vi "Event Handler.vi"(8 "error in (no error)":errorcluster, 10 "Stop Event Handler":refnum<user-event>, 11 "BreadcrumbNavigation in":refnum<class "BreadcrumbNavigator.lvclass">) -> (0 "error out":errorcluster)   [LabVIEW 2015, in "BreadcrumbNavigator.lvclass"]
doc: "The <b>Event Handler VI</b> is a dynamic dispatch VI that should be overwritten if events are needed to create the enhanced QControl. \n\nBy inheriting from the main Control.lvclass the overwritten <b>Event Handler VI</b> will be launched asynchronously in the initialization of the QControl.\n<b> </b> <b> </b>\n©2016 Q Software Innovations, LLC (QSI)\nwritten by Quentin Alldredge\nproduced in LabVIEW 2015\n\nsupport@qsoftwareinnovations.com\nwww.qsoftwareinnovations.com\n\nAll rights reserved.\n\nRedistribution and use in source and binary forms, with or without modification, are permitted provided that the following conditions are met:\n\n * Redistributions of source code must retain the above copyright notice, this list of conditions and the following disclaimer.\n * Redistributions in binary form must reproduce the above copyright notice, this list of conditions and the following disclaimer in the documentation and/or other materials provided with the distribution.\n * Neither the name of Q Software Innovations, LLC. nor the names of its contributors may be used to endorse or promote products derived from this software without specific prior written permission.\n\nTHIS SOFTWARE IS PROVIDED BY THE COPYRIGHT HOLDERS AND CONTRIBUTORS \"AS IS\" AND ANY EXPRESS OR IMPLIED WARRANTIES, INCLUDING, BUT NOT LIMITED TO, THE IMPLIED WARRANTIES OF MERCHANTABILITY AND FITNESS FOR A PARTICULAR PURPOSE ARE DISCLAIMED. IN NO EVENT SHALL THE COPYRIGHT OWNER OR CONTRIBUTORS BE LIABLE FOR ANY DIRECT, INDIRECT, INCIDENTAL, SPECIAL, EXEMPLARY, OR CONSEQUENTIAL DAMAGES (INCLUDING, BUT NOT LIMITED TO, PROCUREMENT OF SUBSTITUTE GOODS OR SERVICES; LOSS OF USE, DATA, OR PROFITS; OR BUSINESS INTERRUPTION) HOWEVER CAUSED AND ON ANY THEORY OF LIABILITY, WHETHER IN CONTRACT, STRICT LIABILITY, OR TORT (INCLUDING NEGLIGENCE OR OTHERWISE) ARISING IN ANY WAY OUT OF THE USE OF THIS SOFTWARE, EVEN IF ADVISED OF THE POSSIBILITY OF SUCH DAMAGE."
uses:
  BreadcrumbNavigator.lvclass
  <vilib>/Utility/cursorutil.llb/Set Cursor (Icon Pict).vi
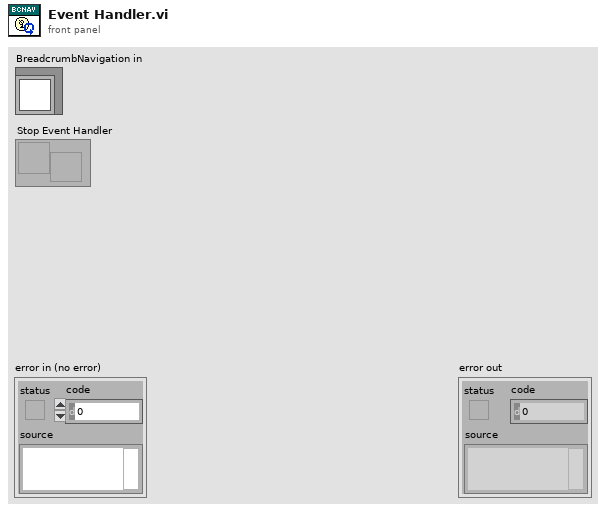
[diagram p1: front panel]
types:
  T1 = typedef "LVPoint32TypeDef.ctl" = cluster{"Horizontal":i32, "Vertical":i32}
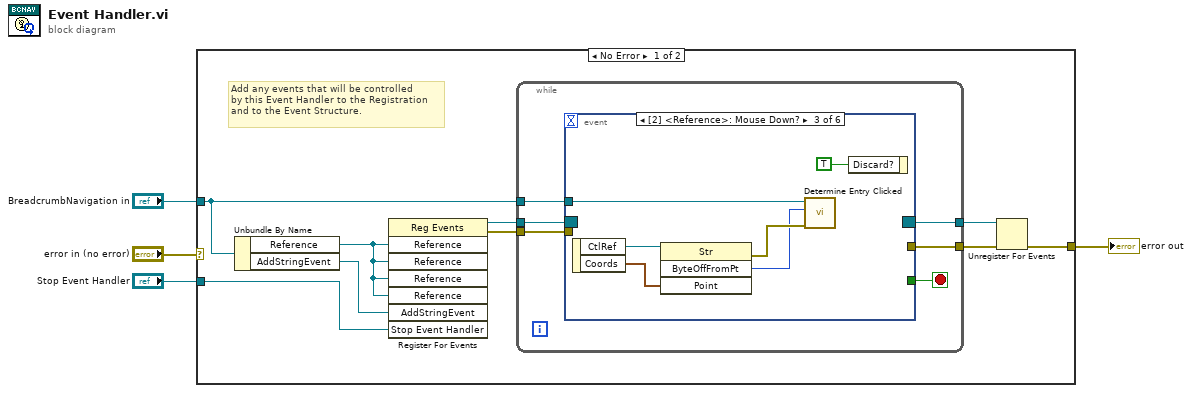
[diagram p0: block diagram]
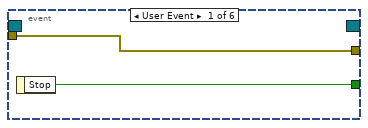
[diagram p2: hidden frame]
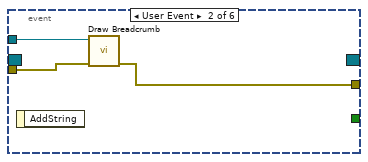
[diagram p3: hidden frame]
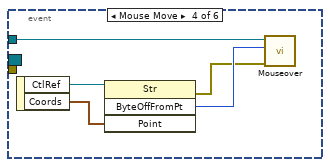
[diagram p4: hidden frame]
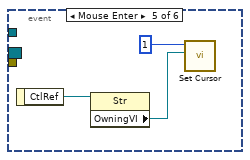
[diagram p5: hidden frame]
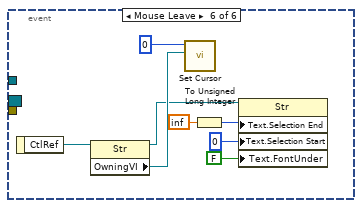
[diagram p6: hidden frame]
diagram:
  n1 = case shown="No Error" "error in (no error)" {
    selector: "error in (no error)" -> [_ w47]
    tunnel: [w10 w47] -> w3
    tunnel: "BreadcrumbNavigation in" -> [w8 _]
    tunnel: "Stop Event Handler" -> [w7 _]
    frame No Error {
      # "Add any events that will be controlled\nby this Event Handler to the Registration\nand to the Event Structure."
      n2 = Unbundle By Name(w8) -> ("Reference"=w5:refnum<vi>, "AddStringEvent"=w6:refnum<user-event>)
      n3 = register-events(w5, w5, w5, w5, w6, w7) -> (reference out=w13:refnum<event-registration>, error out=w12:errorcluster)  [unwired: 2 in]
      n4 = while {
        tunnel: w13 -> [w19]
        tunnel: w12 -> [w17]
        tunnel: [w16] -> w11
        tunnel: [w14] -> w9
        tunnel: w8 -> [w18]
        stop <- w15 stop-if-true
        n5 = event shown="[2] <Reference>: Mouse Down?" {
          selector: w19 -> [_ _ _ _ _ _]
          dyn-events: [_ _ _ _ _ _] -> w14
          timeout: _ -> [_ _ _ _ _ _]
          tunnel: w18 -> [_ w24 w27 w33 _ _]
          tunnel: w17 -> [w21 w23 _ _ _ _]
          tunnel: [w21 w22 _ _ _ _] -> w16
          tunnel: [w20 _ _ _ _ _] -> w15
          event User Event {
            n6 = event-data() -> ("Stop"=w20:bool)  [unwired: 1 in]
          }
          event User Event {
            n7 = event-data() -> ()  [unwired: 1 in, 1 out]
            n8 = call "Draw Breadcrumb.vi"("error in (no error)"=w23, "BreadcrumbNavigation in"=w24) -> ("error out"=w22:errorcluster)  [unwired: 8 in, 1 out]
          }
          event Mouse Down? {
            n9 = event-data() -> ("CtlRef"=w30:refnum<vi>, "Coords"=w29:T1)  [unwired: 1 in]
            n10 = invoke class="Str" method="ByteOffFromPt"(reference=w30, "Point"=w29) -> (error out=w28:errorcluster, "ByteOffFromPt"=w26:i32)  [unwired: 2 in, 2 out]
            n11 = call "Determine Entry Clicked.vi"("error in (no error)"=w28, "Byte Position"=w26, "BreadcrumbNavigation in"=w27) -> ()  [unwired: 7 in, 2 out]
            n12 = event-data("Discard?"=TRUE) -> ()  [unwired: 1 in, 1 out]
          }
          event Mouse Move {
            n13 = event-data() -> ("CtlRef"=w35:refnum<vi>, "Coords"=w34:T1)  [unwired: 1 in]
            n14 = invoke class="Str" method="ByteOffFromPt"(reference=w35, "Point"=w34) -> (error out=w31:errorcluster, "ByteOffFromPt"=w32:i32)  [unwired: 2 in, 2 out]
            n15 = call "Mouseover.vi"("error in (no error)"=w31, "Byte Position"=w32, "BreadcrumbNavigation in"=w33) -> ()  [unwired: 7 in, 2 out]
          }
          event Mouse Enter {
            n16 = event-data() -> ("CtlRef"=w38:refnum<vi>)  [unwired: 1 in]
            n17 = property class="Str"(reference=w38) -> ("OwningVI"=w37:refnum<vi>)  [unwired: 1 in, 2 out]
            n18 = call-poly <vilib>:"Set Cursor.vi"("VI reference (current VI)"=w37, "icon"=u16 1) -> ()  [unwired: 8 in, 2 out]
          }
          event Mouse Leave {
            n19 = event-data() -> ("CtlRef"=w46:refnum<vi>)  [unwired: 1 in]
            n20 = property class="Str"(reference=w46) -> (reference out=w39:refnum<vi>, "OwningVI"=w45:refnum<vi>)  [unwired: 1 in, 1 out]
            n21 = call-poly <vilib>:"Set Cursor.vi"("VI reference (current VI)"=w45, "icon"=u16 0) -> ()  [unwired: 8 in, 2 out]
            n22 = To Unsigned Long Integer(number=inf) -> (unsigned 32bit integer=w43:u32)
            n23 = property class="Str"(reference=w39, "Text.Selection End"=w43, "Text.Selection Start"=u32 0 ("Text.Selection:Start"), "Text.FontUnder"=FALSE ("Text.Font:Underline")) -> ()  [unwired: 1 in, 2 out]
          }
        }
      }
      n24 = Unregister For Events(event registration refnum=w9, error in=w11) -> (error out=w10:errorcluster)
    }
    frame Error {
    }
  }
  "error out" <- w3
